vi "updateDisabledList.vi"(8 "error in (no error)":errorcluster, 11 "ILCCommunications in":refnum<class "ILCCommunications.lvclass">) -> (0 "error out":errorcluster, 3 "ILCCommunications out":refnum<class "ILCCommunications.lvclass">)   [LabVIEW 2016, in "ILCCommunications.lvclass"]
uses:
  ILCCommunications.lvclass
  ILCCommunications.lvclass/ILCCommunications.ctl
  Common_RT_Modbus/ModbusBuffer/ModbusBuffer.lvclass/ModbusBuffer.ctl
  Common_RT_FAILC/FAILC/FAILC.lvclass/FAILC.ctl
  Common_RT_HPILC/HPILC/HPILC.lvclass/HPILC.ctl
  Common_RT_FAILC/FAILC/addBroadcastFreezeSensorValuesFrame.vi
  Common_RT_HPILC/HPILC/addBroadcastFreezeSensorValuesFrame.vi
  Common_RT_Modbus/ModbusBuffer/writeHeader.vi
  Common_RT_Modbus/ModbusBuffer/writeU8.vi
  Common_RT_Modbus/ModbusBuffer/writeCRC.vi
  Common_RT_Modbus/ModbusBuffer/writeEndOfFrame.vi
  Common_RT_Modbus/ModbusBuffer/writeDelay.vi
  Common_RT_Modbus/ModbusBuffer/writeByteInstruction.vi
  Common_RT_Modbus/ModbusBuffer/calculateCRC.vi
  Common_RT_Modbus/ModbusBuffer/ModbusBuffer.lvclass
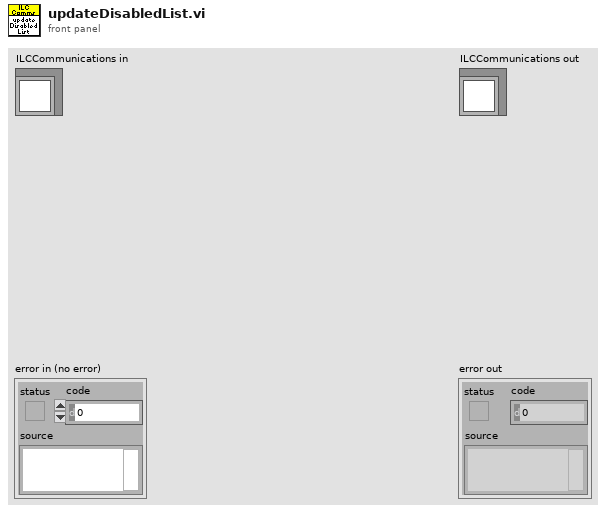
[diagram p1: front panel]
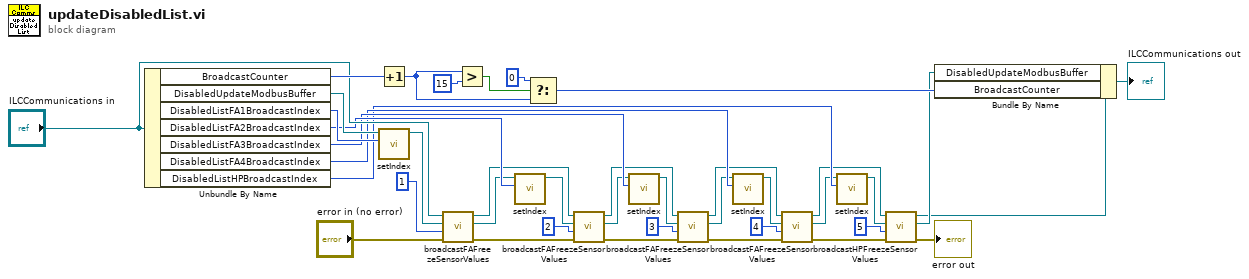
[diagram p0: block diagram]
diagram:
  n1 = Unbundle By Name("ILCCommunications in") -> ("BroadcastCounter"=w39:u8, "DisabledUpdateModbusBuffer"=w40:refnum<class "ModbusBuffer.lvclass">, "DisabledListFA1BroadcastIndex"=w32:i32, "DisabledListFA2BroadcastIndex"=w29:i32, "DisabledListFA3BroadcastIndex"=w23:i32, "DisabledListFA4BroadcastIndex"=w22:i32, "DisabledListHPBroadcastIndex"=w21:i32)
  n2 = Increment(x=w39) -> (x+1=w36:u8)
  n3 = call "setIndex.vi"("Index"=w32, "ModbusBuffer in"=w40) -> ("ModbusBuffer out"=w31:refnum<class "ModbusBuffer.lvclass">)  [unwired: 9 in]
  n4 = call "broadcastFAFreezeSensorValues.vi"("error in (no error)"="error in (no error)", "Subnet"=u8 1, "ModbusBuffer in"=w31, "ILCCommunications in"="ILCCommunications in") -> ("error out"=w24:errorcluster, "ModbusBuffer out"=w27:refnum<class "ModbusBuffer.lvclass">, "ILCCommunications out"=w9:refnum<class "ILCCommunications.lvclass">)  [unwired: 5 in]
  n5 = Greater?(x=w36, y=u8 15) -> (0:w37:bool)
  n6 = call "setIndex.vi"("Index"=w29, "ModbusBuffer in"=w27) -> ("ModbusBuffer out"=w26:refnum<class "ModbusBuffer.lvclass">)  [unwired: 9 in]
  n7 = Select(t=u8 0, s=w37, f=w36) -> (s? t:f=w34:u8)
  n8 = call "broadcastFAFreezeSensorValues.vi"("error in (no error)"=w24, "Subnet"=u8 2, "ModbusBuffer in"=w26, "ILCCommunications in"=w9) -> ("error out"=w13:errorcluster, "ModbusBuffer out"=w20:refnum<class "ModbusBuffer.lvclass">, "ILCCommunications out"=w8:refnum<class "ILCCommunications.lvclass">)  [unwired: 5 in]
  n9 = call "setIndex.vi"("Index"=w23, "ModbusBuffer in"=w20) -> ("ModbusBuffer out"=w19:refnum<class "ModbusBuffer.lvclass">)  [unwired: 9 in]
  n10 = call "broadcastFAFreezeSensorValues.vi"("error in (no error)"=w13, "Subnet"=u8 3, "ModbusBuffer in"=w19, "ILCCommunications in"=w8) -> ("error out"=w12:errorcluster, "ModbusBuffer out"=w18:refnum<class "ModbusBuffer.lvclass">, "ILCCommunications out"=w7:refnum<class "ILCCommunications.lvclass">)  [unwired: 5 in]
  n11 = call "setIndex.vi"("Index"=w22, "ModbusBuffer in"=w18) -> ("ModbusBuffer out"=w17:refnum<class "ModbusBuffer.lvclass">)  [unwired: 9 in]
  n12 = call "broadcastFAFreezeSensorValues.vi"("error in (no error)"=w12, "Subnet"=u8 4, "ModbusBuffer in"=w17, "ILCCommunications in"=w7) -> ("error out"=w3:errorcluster, "ModbusBuffer out"=w16:refnum<class "ModbusBuffer.lvclass">, "ILCCommunications out"=w6:refnum<class "ILCCommunications.lvclass">)  [unwired: 5 in]
  n13 = call "setIndex.vi"("Index"=w21, "ModbusBuffer in"=w16) -> ("ModbusBuffer out"=w11:refnum<class "ModbusBuffer.lvclass">)  [unwired: 9 in]
  n14 = call "broadcastHPFreezeSensorValues.vi"("error in (no error)"=w3, "Subnet"=u8 5, "ModbusBuffer in"=w11, "ILCCommunications in"=w6) -> ("error out"=→"error out":errorcluster, "ModbusBuffer out"=w10:refnum<class "ModbusBuffer.lvclass">, "ILCCommunications out"=w5:refnum<class "ILCCommunications.lvclass">)  [unwired: 5 in]
  n15 = Bundle By Name(cluster=w5, "DisabledUpdateModbusBuffer"=w10, "BroadcastCounter"=w34) -> (→"ILCCommunications out":refnum<class "ILCCommunications.lvclass">)
